vi "Write test data to nimbelink upload file.vi"(4 "Style":string, 5 "Pass date time":string, 6 "error in (no error)":errorcluster, 7 "imei":string, 8 "Meid":string, 9 "Serial Number":string) -> (0 "error out":errorcluster, 2 "PassFail":string, 3 "Write OK?":bool)   [LabVIEW 2013]
uses:
  Test Globals/Global 1.vi
  Main Support/Global 2.vi
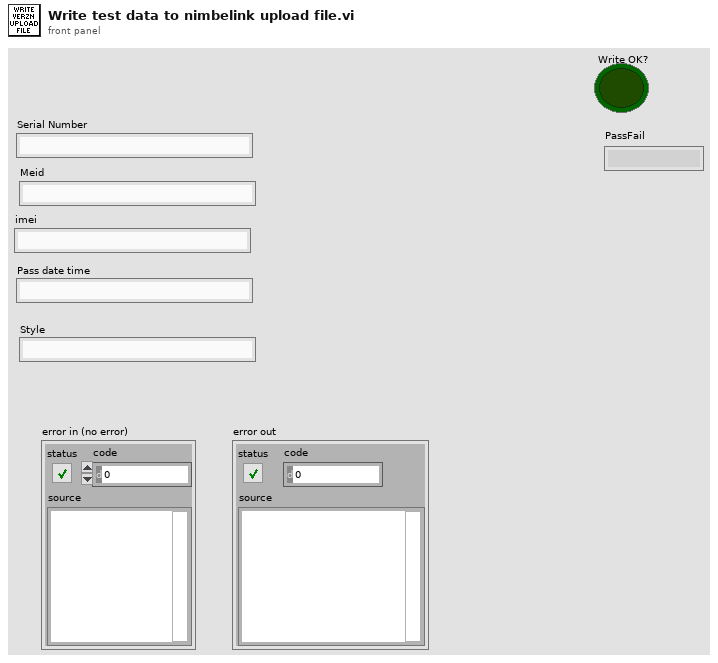
[diagram p1: front panel]
types:
  T1 = cluster{"Test folder":string, "Top level":string, "Main":string, "Test report":string, "Work order qty":string, "Work order meid":string, "Work order imei":string, "Master meid imei list":string, "Master test data":string, "ZPL label info":string, "Pictures":string, "Setup info":string, "Work order":string, "Tests folder":string, "Tests steps folder":string, "Config folder":string, "Verizon Upload file":string, "Job data file":string, "Station globals":string, "Post test info":string}
  T2 = enum16{"open", "replace", "create", "open or create", "replace or create", "replace or create with confirmation"}
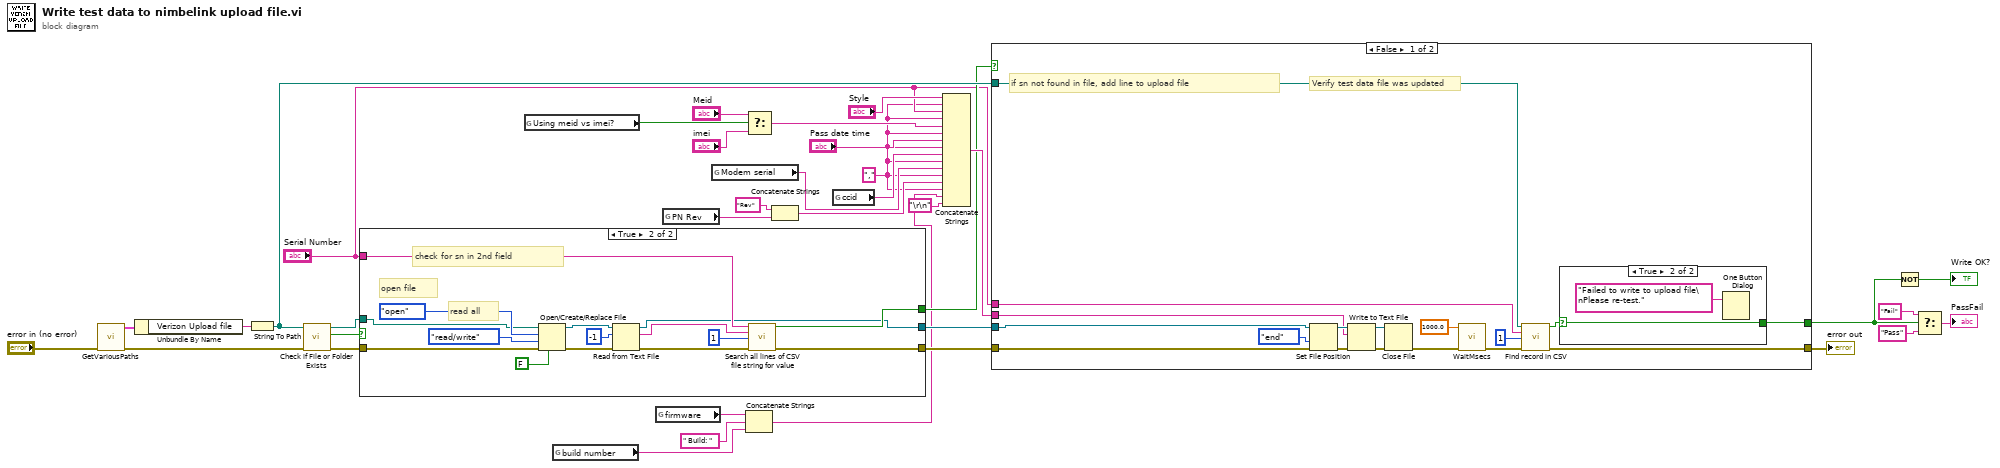
[diagram p0: block diagram]
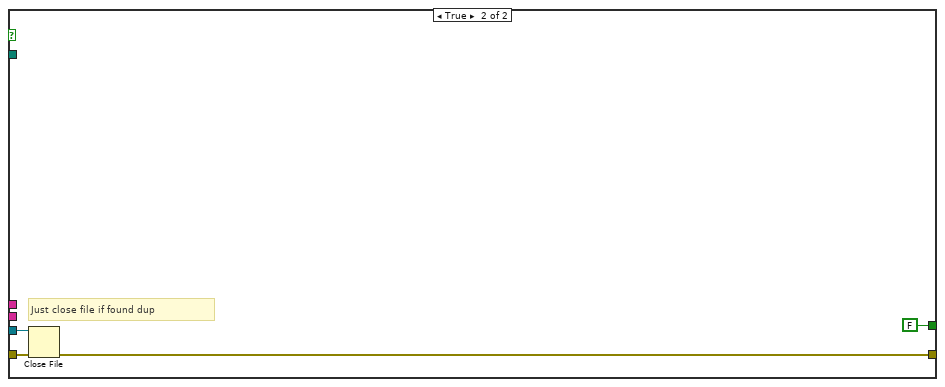
[diagram p3: hidden frame]
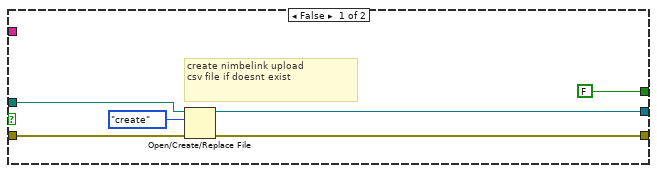
[diagram p4: hidden frame]
diagram:
  w1 = "," ("string")
  n1 = call "GetVariousPaths.vi"("error in (no error)"="error in (no error)") -> ("error out"=w26:errorcluster, "Built Paths"=w33:T1)  [unwired: 9 in]
  n2 = Unbundle By Name(w33) -> ("Verizon Upload file"=w34:string)
  n3 = String To Path(string=w34) -> (path=w25:path)
  n4 = call <vilib>:"Check if File or Folder Exists.vi"("error in (no error)"=w26, "path"=w25) -> ("error out"=w22:errorcluster, "file or folder exists?"=w24:bool, "dup path"=w23:path)  [unwired: 7 in]
  n5 = case shown="True" w24 {
    tunnel: w23 -> [w41 w54]
    tunnel: w22 -> [w40 w53]
    tunnel: [w39 w45] -> w17
    tunnel: "Serial Number" -> [_ w47]
    tunnel: [FALSE ("Found value") w44] -> w16
    tunnel: [w38 w43] -> w15
    frame False {
      # "create nimbelink upload\ncsv file if doesnt exist"
      n6 = Open/Create/Replace File(file path (use dialog)=w41, error in=w40, operation (0:open)=T2."create") -> (refnum out=w38:refnum<file>, error out=w39:errorcluster)  [unwired: 3 in, 1 out]
    }
    frame True {
      # "check for sn in 2nd field"
      # "read all"
      # "open file"
      n7 = Open/Create/Replace File(file path (use dialog)=w54, error in=w53, operation (0:open)=T2."open", access (0:read/write)=enum16{"read/write", "read-only", "write-only"}."read/write", disable buffering (F)=FALSE) -> (refnum out=w51:refnum<file>, error out=w50:errorcluster)  [unwired: 1 in, 1 out]
      n8 = Read from Text File(file (use dialog)=w51, count=-1, error in=w50) -> (refnum out=w43:refnum<file>, text=w48:string, error out=w49:errorcluster)  [unwired: 1 in, 1 out]
      n9 = call "Search all lines of CSV file string for value.vi"("Compare value"=w47, "CSV file string"=w48, "CSV field (0-n)"=1, "error in"=w49) -> ("Found value"=w44:bool, "error out"=w45:errorcluster)  [unwired: 10 in]
    }
  }
  n10 = global read "Global 1.vi" "Using meid vs imei?"() -> (w31:bool)
  n11 = global read "Global 1.vi" "build number"() -> (w2:string)
  n12 = global read "Global 1.vi" "firmware"() -> (w5:string)
  n13 = global read "Global 2.vi" "PN Rev"() -> (w8:string)
  n14 = global read "Global 1.vi" "Modem serial"() -> (w9:string)
  n15 = Concatenate Strings(w5, " Build: " ("string"), w2) -> (w3:string)
  n16 = Select(t="Meid", s=w31, f="imei") -> (s? t:f=w28:string)
  n17 = Concatenate Strings("Rev" ("string"), w8) -> (w6:string)
  n18 = global read "Global 1.vi" "ccid"() -> (w11:string)
  n19 = Concatenate Strings("Style", w1, "Serial Number", w1, w28, w1, "Pass date time", w1, w11, w1, w9, w1, w6, w1, w3, "\r\n") -> (w18:string)
  n20 = case shown="False" w16 {
    tunnel: [w60 w79] -> w13
    tunnel: w25 -> [w59 _]
    tunnel: w17 -> [w68 w80]
    tunnel: w18 -> [w71 _]
    tunnel: w15 -> [w67 w81]
    tunnel: [w61 FALSE] -> w14
    tunnel: "Serial Number" -> [w58 _]
    frame False {
      # "Verify test data file was updated"
      # "if sn not found in file, add line to upload file"
      n21 = Set File Position(refnum=w67, from (0:start)=enum16{"start", "end", "current"}."end", error in=w68) -> (refnum out=w72:refnum<file>, error out=w73:errorcluster)  [unwired: 1 in]
      n22 = Write to Text File(file (use dialog)=w72, text=w71, error in=w73) -> (refnum out=w69:refnum<file>, error out=w70:errorcluster)  [unwired: 1 in, 1 out]
      n23 = Close File(refnum=w69, error in=w70) -> (error out=w62:errorcluster)  [unwired: 1 out]
      n24 = call "WaitMsecs.vi"("error in (no error)"=w62, "Wait Msecs"=1000.0) -> ("error out"=w64:errorcluster)  [unwired: 9 in]
      n25 = call "Find record in CSV.vi"("CSV file"=w59, "Search key"=w58, "Search key column (0-n)"=u32 1, "error in"=w64) -> ("Record not found?"=w66:bool, "error out"=w60:errorcluster)  [unwired: 3 in, 7 out]
      n26 = case shown="True" w66 {
        selector: w66 -> [w75 w76]
        tunnel: [w75 w76] -> w61
        frame False {
        }
        frame True {
          n27 = One Button Dialog(message="Failed to write to upload file\nPlease re-test.") -> ()  [unwired: 1 in, 1 out]
        }
      }
    }
    frame True {
      # "Just close file if found dup"
      n28 = Close File(refnum=w81, error in=w80) -> (error out=w79:errorcluster)  [unwired: 1 out]
    }
  }
  "error out" <- w13
  n29 = Not(x=w14) -> (.not. x?=→"Write OK?":bool)
  n30 = Select(t="Fail" ("message"), s=w14, f="Pass" ("message")) -> (s? t:f=→"PassFail":string)
